vi "setChannelDefaultValues.vi"(8 "error in (no error)":errorcluster, 9 "calibratedValues":dbl[](array[numeric]), 10 "channel_addresses":string[](array[string]), 11 "DigitalOutput in":refnum<class "DigitalOutput.lvclass">) -> (0 "error out":errorcluster, 3 "DigitalOutput out":refnum<class "DigitalOutput.lvclass">)   [LabVIEW 2009, in "Hardware.lvlib" / "Channels.lvlib" / "DigitalOutput.lvclass"]
uses:
  DigitalOutput.lvclass
  DigitalOutput.lvclass/DigitalOutput.ctl
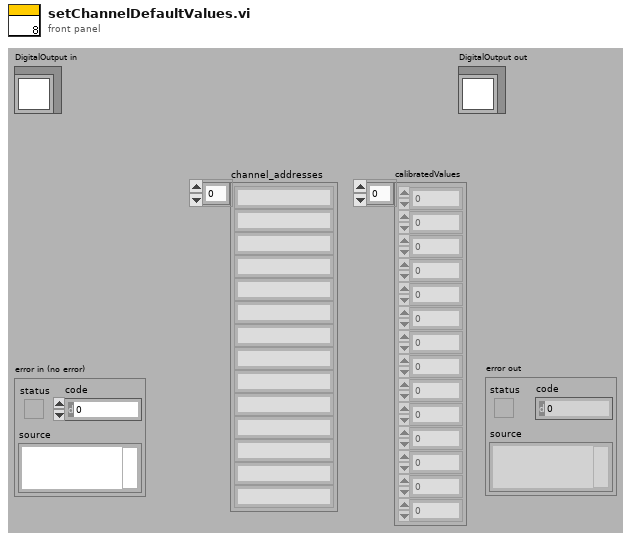
[diagram p1: front panel]
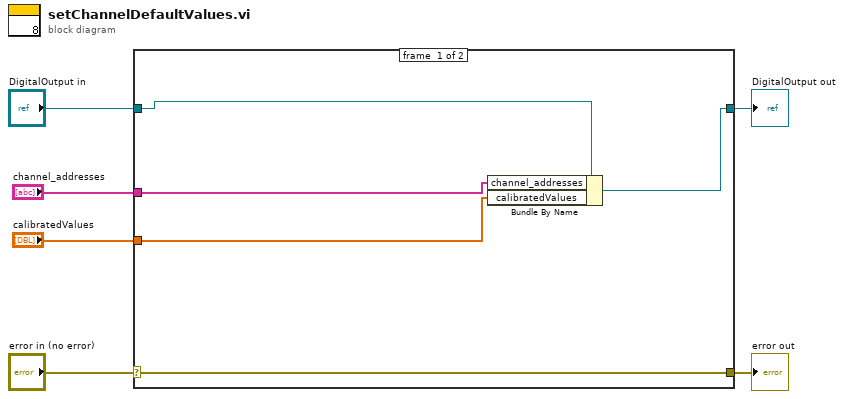
[diagram p0: block diagram]
diagram:
  n1 = case shown="No Error" "error in (no error)" {
    selector: "error in (no error)" -> [w11 w13]
    tunnel: [w11 w13] -> w5
    tunnel: [w9 w12] -> w3
    tunnel: "DigitalOutput in" -> [w10 w12]
    tunnel: "channel_addresses" -> [w8 _]
    tunnel: "calibratedValues" -> [w7 _]
    frame #0 {
      n2 = Bundle By Name(cluster=w10, "channel_addresses"=w8, "calibratedValues"=w7) -> (w9:refnum<class "DigitalOutput.lvclass">)
    }
    frame #1 {
    }
  }
  "error out" <- w5
  "DigitalOutput out" <- w3
